vi "OE2011&OE2021_DATA Transmit.vi"(5 "Input Data":u8[](array[numeric])) -> (0 "Trig_Count":u8[](array[numeric]), 1 "PLL&Overload":T2, 2 "Parameter Values":T1, 3 "Total Date Array":dbl[][](array[numeric]), 4 "Buffer Count":u8)   [LabVIEW 2011]
panel:
  out "θh8":dbl[](array[numeric])
  out "Rh8":dbl[](array[numeric])
  out "θh7":dbl[](array[numeric])
  out "Rh7":dbl[](array[numeric])
  out "θh6":dbl[](array[numeric])
  out "Rh6":dbl[](array[numeric])
  out "θh5":dbl[](array[numeric])
  out "Rh5":dbl[](array[numeric])
  out "θh4":dbl[](array[numeric])
  out "Rh4":dbl[](array[numeric])
  out "θh3":dbl[](array[numeric])
  out "Rh3":dbl[](array[numeric])
  out "θh2":dbl[](array[numeric])
  out "Rh2":dbl[](array[numeric])
  out "θh1":dbl[](array[numeric])
  out "Rh1":dbl[](array[numeric])
  out "Osc1_Freq":dbl[](array[numeric])
  out "AUX IN2":dbl[](array[numeric])
  out "Yh8_Noise":dbl[](array[numeric])
  out "AUX IN1":dbl[](array[numeric])
  out "Osc2_Freq":dbl[](array[numeric])
  out "Xh8_Noise":dbl[](array[numeric])
  out "Yh6":dbl[](array[numeric])
  out "Yh5_Noise":dbl[](array[numeric])
  out "Xh6_Noise":dbl[](array[numeric])
  out "Yh6_Noise":dbl[](array[numeric])
  out "Xh7_Noise":dbl[](array[numeric])
  out "Yh7_Noise":dbl[](array[numeric])
  out "Xh6":dbl[](array[numeric])
  out "Xh7":dbl[](array[numeric])
  out "Yh7":dbl[](array[numeric])
  out "Xh8":dbl[](array[numeric])
  out "Yh8":dbl[](array[numeric])
  out "Xh1":dbl[](array[numeric])
  out "Yh1":dbl[](array[numeric])
  out "Xh2_Noise":dbl[](array[numeric])
  out "Xh2":dbl[](array[numeric])
  out "Yh2_Noise":dbl[](array[numeric])
  out "Xh3":dbl[](array[numeric])
  out "Yh3_Noise":dbl[](array[numeric])
  out "Xh4":dbl[](array[numeric])
  out "AUX IN3":dbl[](array[numeric])
  out "AUX IN4":dbl[](array[numeric])
  out "Yh4_Noise":dbl[](array[numeric])
  out "Xh5":dbl[](array[numeric])
  out "Yh2":dbl[](array[numeric])
  out "Xh1_Noise":dbl[](array[numeric])
  out "Yh1_Noise":dbl[](array[numeric])
  out "Yh3":dbl[](array[numeric])
  out "Xh3_Noise":dbl[](array[numeric])
  out "Yh4":dbl[](array[numeric])
  out "Xh4_Noise":dbl[](array[numeric])
  out "Yh5":dbl[](array[numeric])
  out "Xh5_Noise":dbl[](array[numeric])
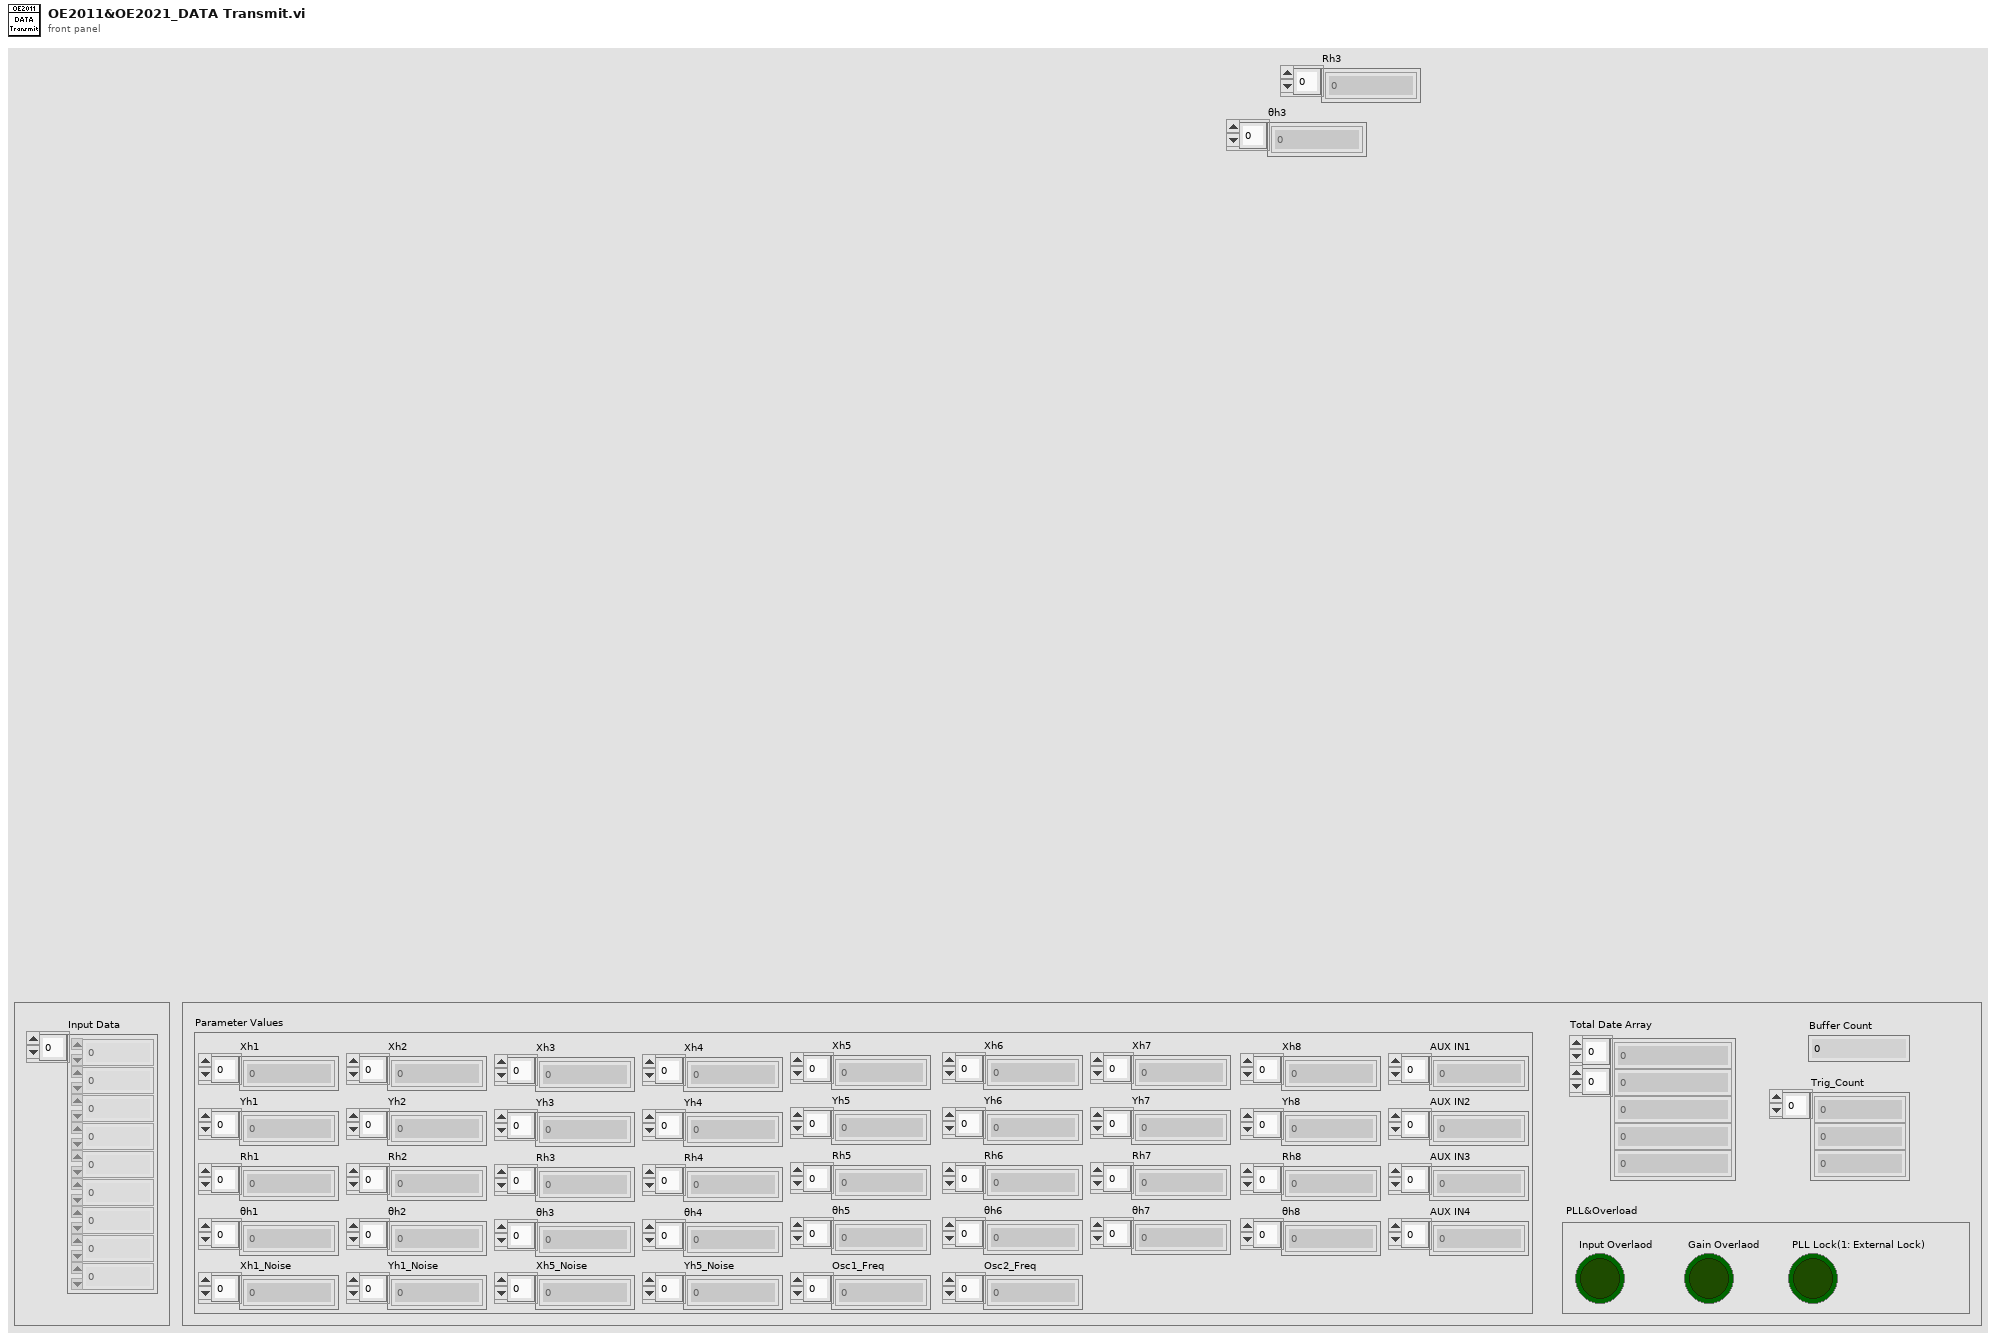
[diagram p1: front panel]
types:
  T1 = cluster{"Xh1":dbl[], "Yh1":dbl[], "Rh1":dbl[], "θh1":dbl[], "Xh1_Noise":dbl[], "Yh1_Noise":dbl[], "Xh2":dbl[], "Yh2":dbl[], "Rh2":dbl[], "θh2":dbl[], "Xh3":dbl[], "Yh3":dbl[], "Rh3":dbl[], "θh3":dbl[], "Xh4":dbl[], "Yh4":dbl[], "Rh4":dbl[], "θh4":dbl[], "Xh5":dbl[], "Yh5":dbl[], "Rh5":dbl[], "θh5":dbl[], "Xh5_Noise":dbl[], "Yh5_Noise":dbl[], "Xh6":dbl[], "Yh6":dbl[], "Rh6":dbl[], "θh6":dbl[], "Xh7":dbl[], "Yh7":dbl[], "Rh7":dbl[], "θh7":dbl[], "Xh8":dbl[], "Yh8":dbl[], "Rh8":dbl[], "θh8":dbl[], "Osc1_Freq":dbl[], "Osc2_Freq":dbl[], "AUX IN1":dbl[], "AUX IN2":dbl[], "AUX IN3":dbl[], "AUX IN4":dbl[]}
  T2 = cluster{"Input Overlaod":bool, "Gain Overlaod":bool, "PLL Lock(1: External Lock)":bool}
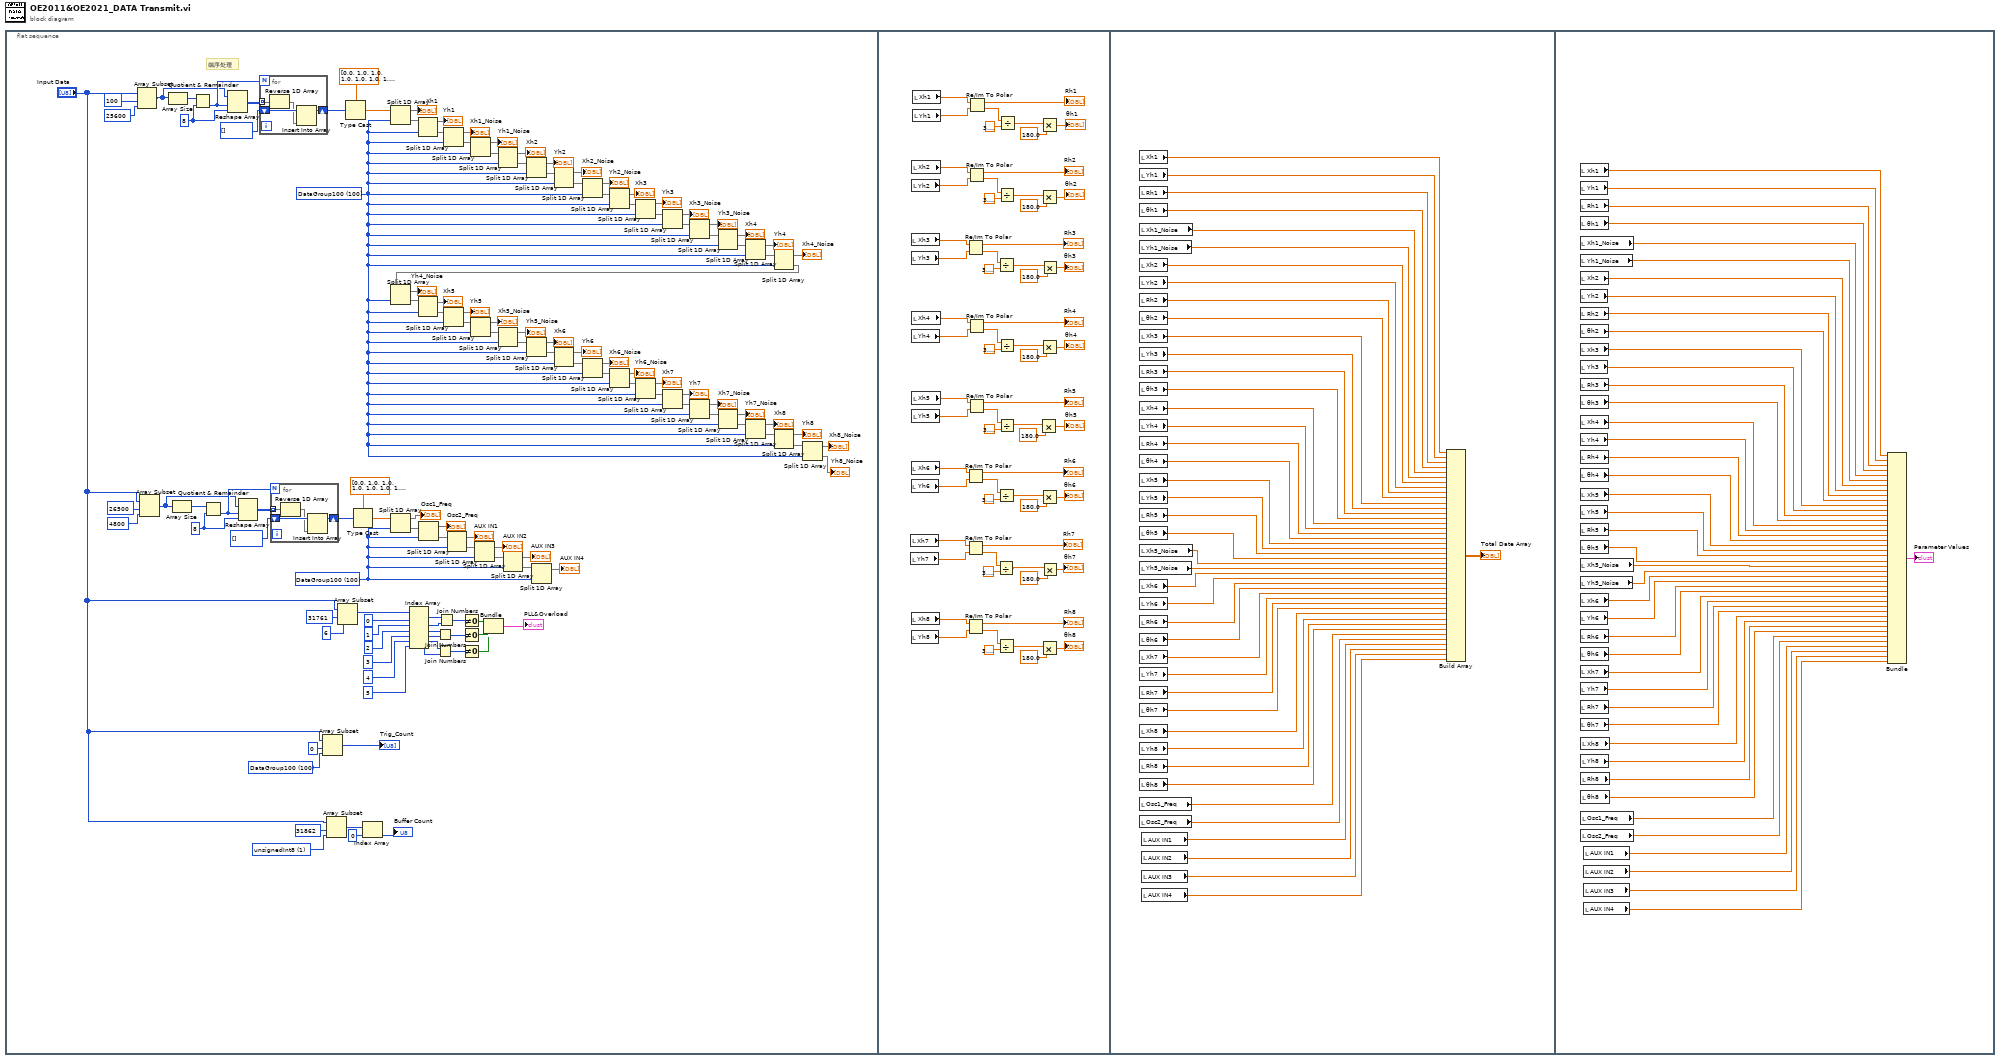
[diagram p0: block diagram]
diagram:
  n1 = flat-sequence {
    frame #0 {
      w5 = u16 1 items=["unsignedInt8"=1, "unsignedInt16"=2, "unsignedInt32"=4, "unsignedInt64"=8, "Float"=80, "Double"=160, "StartLength"=2240, "DataGroup50"=50, "DataGroup100"=100, "DataGroup20"=20] ("数据类型")
      w25 = 8 ("y")
      w30 = 8 ("y")
      w35 = u16 100 items=["unsignedInt8"=1, "unsignedInt16"=2, "unsignedInt32"=4, "unsignedInt64"=8, "Float"=80, "Double"=160, "StartLength"=2240, "DataGroup50"=50, "DataGroup100"=100, "DataGroup20"=20] ("数据类型")
      w46 = u16 100 items=["unsignedInt8"=1, "unsignedInt16"=2, "unsignedInt32"=4, "unsignedInt64"=8, "Float"=80, "Double"=160, "StartLength"=2240, "DataGroup50"=50, "DataGroup100"=100, "DataGroup20"=20] ("数据类型")
      w54 = u16 100 items=["unsignedInt8"=1, "unsignedInt16"=2, "unsignedInt32"=4, "unsignedInt64"=8, "Float"=80, "Double"=160, "StartLength"=2240, "DataGroup50"=50, "DataGroup100"=100, "DataGroup20"=20] ("数据类型")
      # "端序处理"
      n2 = Array Subset(array="Input Data", index=100 ("索引"), length=25600 ("长度")) -> (w22:u8[])
      n3 = Array Subset(array="Input Data", index=26500 ("索引"), length=4800 ("长度")) -> (w21:u8[])
      n4 = Array Size(array=w22) -> (size(s)=w29:i32)
      n5 = Array Size(array=w21) -> (size(s)=w24:i32)
      n6 = Quotient & Remainder(x=w29, y=w30) -> (floor(x/y)=w32:i32)  [unwired: 1 out]
      n7 = Quotient & Remainder(x=w24, y=w25) -> (floor(x/y)=w27:i32)  [unwired: 1 out]
      n8 = Reshape Array(w22, w32, w30) -> (w31:u8[][])
      n9 = Reshape Array(w21, w27, w25) -> (w26:u8[][])
      n10 = for {
        N: w32 -> [_]
        tunnel: w31 -> [w136] mode=indexing
        shift-right: [w134] -> w20
        shift-left: u8[] [] -> [w135]
        n11 = Reverse 1D Array(array=w136) -> (reversed array=w133:u8[])
        n12 = Insert Into Array(array=w135, new element=w133) -> (w134:u8[])  [unwired: 1 in]
      }
      n13 = for {
        N: w27 -> [_]
        tunnel: w26 -> [w132] mode=indexing
        shift-right: [w130] -> w23
        shift-left: u8[] [] -> [w131]
        n14 = Reverse 1D Array(array=w132) -> (reversed array=w129:u8[])
        n15 = Insert Into Array(array=w131, new element=w129) -> (w130:u8[])  [unwired: 1 in]
      }
      n16 = Array Subset(array="Input Data", index=0 ("索引"), length=w46) -> (→"Trig_Count":u8[])
      n17 = Array Subset(array="Input Data", index=31862 ("索引"), length=w5) -> (w3:u8[])
      n18 = Array Subset(array="Input Data", index=31761 ("索引"), length=6 ("长度")) -> (w51:u8[])
      n19 = Type Cast(type=dbl[] [0.0, 1.0, 1.0, 1.0, 1.0, 1.0, 1.0, 1.0, 1.0, 1.0, 1.0, 1.0, 1.0, 1.0, 1.0, 1.0, 1.0, 1.0, 1.0, 1.0, 1.0, 1.0, 1.0, 1.0, 1.0, 1.0, 1.0, 1.0, 1.0, 1.0, 1.0, 1.0, 1.0, 1.0, 1.0, 1.0, 1.0, 1.0, 1.0, 1.0, 1.0, 1.0, 1.0, 1.0, 1.0, 1.0, 1.0, 1.0, 1.0, 1.0, 1.0, 1.0, 1.0, 1.0, 1.0, 1.0, 1.0, 1.0, 1.0, 1.0, 1.0, 1.0, 1.0, 1.0, 1.0, 1.0, 1.0, 1.0, 1.0, 1.0, 1.0, 1.0, 1.0, 1.0, 1.0, 1.0, 1.0, 1.0, 1.0, 1.0, 1.0, 1.0, 1.0, 1.0, 1.0, 1.0, 1.0, 1.0, 1.0, 1.0, 1.0, 1.0, 1.0, 1.0, 1.0, 1.0, 1.0, 1.0, 1.0, 1.0, 1.0, 1.0, 1.0, 1.0, 1.0, 1.0, 1.0, 1.0, 1.0, 1.0, 1.0, 1.0, 1.0, 1.0, 1.0, 1.0, 1.0, 1.0, 1.0, 1.0, 1.0, 1.0, 1.0, 1.0, 1.0, 1.0, 1.0, 1.0, 1.0, 1.0, 1.0, 1.0, 1.0, 1.0, 1.0, 1.0, 1.0, 1.0, 1.0, 1.0, 1.0, 1.0, 1.0, 1.0, 1.0, 1.0, 1.0, 1.0, 1.0, 1.0, 1.0, 1.0, 1.0, 1.0, 1.0, 1.0, 1.0, 1.0, 1.0, 1.0, 1.0, 1.0, 1.0, 1.0, 1.0, 1.0, 1.0, 1.0, 1.0, 1.0, 1.0, 1.0, 1.0, 1.0, 1.0, 1.0, 1.0, 1.0, 1.0, 1.0, 1.0, 1.0, 1.0, 1.0, 1.0, 1.0, 1.0, 1.0, 1.0, 1.0, 1.0, 1.0, 1.0, 1.0, 1.0, 1.0, 1.0, 1.0, 1.0, 1.0, 1.0, 1.0, 1.0, 1.0, 1.0, 1.0, 1.0, 1.0, 1.0, 1.0, 1.0, 1.0, 1.0, 1.0, 1.0, 1.0, 1.0, 1.0, 1.0, 1.0, 1.0, 1.0, 1.0, 1.0, 1.0, 1.0, 1.0, 1.0, 1.0, 1.0, 1.0, 1.0, 1.0, 1.0, 1.0, 1.0, 1.0, 1.0, 1.0, 1.0, 1.0, 1.0, 1.0, 1.0, 1.0, 1.0, 1.0, 1.0, 1.0, 1.0, 1.0, 1.0, 1.0, 1.0, 1.0, 1.0, 1.0, 1.0, 1.0, 1.0, 1.0, 1.0, 1.0, 1.0, 1.0, 1.0, 1.0, 1.0, 1.0, 1.0, 1.0, 1.0, 1.0, 1.0, 1.0, 1.0, 1.0, 1.0, 1.0, 1.0, 1.0, 1.0, 1.0, 1.0, 1.0, 1.0, 1.0, 1.0, 1.0, 1.0, 1.0, 1.0, 1.0, 1.0, 1.0, 1.0, 1.0, 1.0, 1.0, 1.0, 1.0, 1.0, 1.0, 1.0, 1.0, 1.0, 1.0, 1.0, 1.0, 1.0, 1.0, 1.0, 1.0, 1.0, 1.0, 1.0, 1.0, 1.0, 1.0, 1.0, 1.0, 1.0, 1.0, 1.0, 1.0, 1.0, 1.0, 1.0, 1.0, 1.0, 1.0, 1.0, 1.0, 1.0, 1.0, 1.0, 1.0, 1.0, 1.0, 1.0, 1.0, 1.0, 1.0, 1.0, 1.0, 1.0, 1.0, 1.0, 1.0, 1.0, 1.0, 1.0, 1.0, 1.0, 1.0, 1.0, 1.0, 1.0, 1.0, 1.0, 1.0, 1.0, 1.0, 1.0, 1.0, 1.0, 1.0, 1.0, 1.0, 1.0, 1.0, 1.0, 1.0, 1.0, 1.0, 1.0, 1.0, 1.0, 1.0, 1.0, 1.0, 1.0, 1.0, 1.0, 1.0, 1.0, 1.0, 1.0, 1.0, 1.0, 1.0, 1.0, 1.0, 1.0, 1.0, 1.0, 1.0, 1.0, 1.0, 1.0, 0.0, 1.0, 1.0, 1.0, 1.0, 1.0, 1.0, 1.0, 1.0, 1.0, 1.0, 1.0, 1.0, 1.0, 1.0, 1.0, 1.0, 1.0, 1.0, 1.0, 1.0, 1.0, 1.0, 1.0, 1.0, 1.0, 1.0, 1.0, 1.0, 1.0, 1.0, 1.0, 1.0, 1.0, 1.0, 1.0, 1.0, 1.0, 1.0, 1.0, 1.0, 1.0, 1.0, 1.0, 1.0, 1.0, 1.0, 1.0, 1.0, 1.0, 1.0, 1.0, 1.0, 1.0, 1.0, 1.0, 1.0, 1.0, 1.0, 1.0, 1.0, 1.0, 1.0, 1.0, 1.0, 1.0, 1.0, 1.0, 1.0, 1.0, 1.0, 1.0, 1.0, 1.0, 1.0, 1.0, 1.0, 1.0, 1.0, 1.0, 1.0, 1.0, 1.0, 1.0, 1.0, 1.0, 1.0, 1.0, 1.0, 1.0, 1.0, 1.0, 1.0, 1.0, 1.0, 1.0, 1.0, 1.0, 1.0, 1.0, 1.0, 1.0, 1.0, 1.0, 1.0, 1.0, 1.0, 1.0, 1.0, 1.0, 1.0, 1.0, 1.0, 1.0, 1.0, 1.0, 1.0, 1.0, 1.0, 1.0, 1.0, 1.0, 1.0, 1.0, 1.0, 1.0, 1.0, 1.0, 1.0, 1.0, 1.0, 1.0, 1.0, 1.0, 1.0, 1.0, 1.0, 1.0, 1.0, 1.0, 1.0, 1.0, 1.0, 1.0, 1.0, 1.0, 1.0, 1.0, 1.0, 1.0, 1.0, 1.0, 1.0, 1.0, 1.0, 1.0, 1.0, 1.0, 1.0, 1.0, 1.0, 1.0, 1.0, 1.0, 1.0, 1.0, 1.0, 1.0, 1.0, 1.0, 1.0, 1.0, 1.0, 1.0, 1.0, 1.0, 1.0, 1.0, 1.0, 1.0, 1.0, 1.0, 1.0, 1.0, 1.0, 1.0, 1.0, 1.0, 1.0, 1.0, 1.0, 1.0, 1.0, 1.0, 1.0, 1.0, 1.0, 1.0, 1.0, 1.0, 1.0, 1.0, 1.0, 1.0, 1.0, 1.0, 1.0, 1.0, 1.0, 1.0, 1.0, 1.0, 1.0, 1.0, 1.0, 1.0, 1.0, 1.0, 1.0, 1.0, 1.0, 1.0, 1.0, 1.0, 1.0, 1.0, 1.0, 1.0, 1.0, 1.0, 1.0, 1.0, 1.0, 1.0, 1.0, 1.0, 1.0, 1.0, 1.0, 1.0, 1.0, 1.0, 1.0, 1.0, 1.0, 1.0, 1.0, 1.0, 1.0, 1.0, 1.0, 1.0, 1.0, 1.0, 1.0, 1.0, 1.0, 1.0, 1.0, 1.0, 1.0, 1.0, 1.0, 1.0, 1.0, 1.0, 1.0, 1.0, 1.0, 1.0, 1.0, 1.0, 1.0, 1.0, 1.0, 1.0, 1.0, 1.0, 1.0, 1.0, 1.0, 1.0, 1.0, 1.0, 1.0, 1.0, 1.0, 1.0, 1.0, 1.0, 1.0, 1.0, 1.0, 1.0, 1.0, 1.0, 1.0, 1.0, 1.0, 1.0, 1.0, 1.0, 1.0, 1.0, 1.0, 1.0, 1.0, 1.0, 1.0, 1.0, 1.0, 1.0, 1.0, 1.0, 1.0, 1.0, 1.0, 1.0, 1.0, 1.0, 1.0, 1.0, 1.0, 1.0, 1.0, 1.0, 1.0, 1.0, 1.0, 1.0, 1.0, 1.0, 1.0, 1.0, 1.0, 1.0, 1.0, 1.0, 1.0, 1.0, 1.0, 1.0, 1.0, 1.0, 1.0, 1.0, 1.0, 1.0, 1.0, 1.0, 1.0, 1.0, 1.0, 1.0, 1.0, 1.0, 1.0, 1.0, 1.0, 1.0, 1.0, 1.0, 1.0, 1.0, 1.0, 1.0, 1.0, 1.0, 1.0, 1.0, 1.0, 1.0, 1.0, 1.0, 1.0, 1.0, 1.0, 1.0, 1.0, 1.0, 1.0, 1.0, 1.0, 1.0, 1.0, 1.0, 1.0, 1.0, 1.0, 1.0, 1.0, 1.0, 1.0, 1.0, 1.0, 1.0, 1.0, 1.0, 1.0, 1.0], x=w20) -> (*(type *) &x=w125:dbl[])
      n20 = Type Cast(type=dbl[] [0.0, 1.0, 1.0, 1.0, 1.0, 1.0, 1.0, 1.0, 1.0, 1.0, 1.0, 1.0, 1.0, 1.0, 1.0, 1.0, 1.0, 1.0, 1.0, 1.0, 1.0, 1.0, 1.0, 1.0, 1.0, 1.0, 1.0, 1.0, 1.0, 1.0, 1.0, 1.0, 1.0, 1.0, 1.0, 1.0, 1.0, 1.0, 1.0, 1.0, 1.0, 1.0, 1.0, 1.0, 1.0, 1.0, 1.0, 1.0, 1.0, 1.0, 1.0, 1.0, 1.0, 1.0, 1.0, 1.0, 1.0, 1.0, 1.0, 1.0, 1.0, 1.0, 1.0, 1.0, 1.0, 1.0, 1.0, 1.0, 1.0, 1.0, 1.0, 1.0, 1.0, 1.0, 1.0, 1.0, 1.0, 1.0, 1.0, 1.0, 1.0, 1.0, 1.0, 1.0, 1.0, 1.0, 1.0, 1.0, 1.0, 1.0, 1.0, 1.0, 1.0, 1.0, 1.0, 1.0, 1.0, 1.0, 1.0, 1.0, 1.0, 1.0, 1.0, 1.0, 1.0, 1.0, 1.0, 1.0, 1.0, 1.0, 1.0, 1.0, 1.0, 1.0, 1.0, 1.0, 1.0, 1.0, 1.0, 1.0, 1.0, 1.0, 1.0, 1.0, 1.0, 1.0, 1.0, 1.0, 1.0, 1.0, 1.0, 1.0, 1.0, 1.0, 1.0, 1.0, 1.0, 1.0, 1.0, 1.0, 1.0, 1.0, 1.0, 1.0, 1.0, 1.0, 1.0, 1.0, 1.0, 1.0, 1.0, 1.0, 1.0, 1.0, 1.0, 1.0, 1.0, 1.0, 1.0, 1.0, 1.0, 1.0, 1.0, 1.0, 1.0, 1.0, 1.0, 1.0, 1.0, 1.0, 1.0, 1.0, 1.0, 1.0, 1.0, 1.0, 1.0, 1.0, 1.0, 1.0, 1.0, 1.0, 1.0, 1.0, 1.0, 1.0, 1.0, 1.0, 1.0, 1.0, 1.0, 1.0, 1.0, 1.0, 1.0, 1.0, 1.0, 1.0, 1.0, 1.0, 1.0, 1.0, 1.0, 1.0, 1.0, 1.0, 1.0, 1.0, 1.0, 1.0, 1.0, 1.0, 1.0, 1.0, 1.0, 1.0, 1.0, 1.0, 1.0, 1.0, 1.0, 1.0, 1.0, 1.0, 1.0, 1.0, 1.0, 1.0, 1.0, 1.0, 1.0, 1.0, 1.0, 1.0, 1.0, 1.0, 1.0, 1.0, 1.0, 1.0, 1.0, 1.0, 1.0, 1.0, 1.0, 1.0, 1.0, 1.0, 1.0, 1.0, 1.0, 1.0, 1.0, 1.0, 1.0, 1.0, 1.0, 1.0, 1.0, 1.0, 1.0, 1.0, 1.0, 1.0, 1.0, 1.0, 1.0, 1.0, 1.0, 1.0, 1.0, 1.0, 1.0, 1.0, 1.0, 1.0, 1.0, 1.0, 1.0, 1.0, 1.0, 1.0, 1.0, 1.0, 1.0, 1.0, 1.0, 1.0, 1.0, 1.0, 1.0, 1.0, 1.0, 1.0, 1.0, 1.0, 1.0, 1.0, 1.0, 1.0, 1.0, 1.0, 1.0, 1.0, 1.0, 1.0, 1.0, 1.0, 1.0, 1.0, 1.0, 1.0, 1.0, 1.0, 1.0, 1.0, 1.0, 1.0, 1.0, 1.0, 1.0, 1.0, 1.0, 1.0, 1.0, 1.0, 1.0, 1.0, 1.0, 1.0, 1.0, 1.0, 1.0, 1.0, 1.0, 1.0, 1.0, 1.0, 1.0, 1.0, 1.0, 1.0, 1.0, 1.0, 1.0, 1.0, 1.0, 1.0, 1.0, 1.0, 1.0, 1.0, 1.0, 1.0, 1.0, 1.0, 1.0, 1.0, 1.0, 1.0, 1.0, 1.0, 1.0, 1.0, 1.0, 1.0, 1.0, 1.0, 1.0, 1.0, 1.0, 1.0, 1.0, 1.0, 1.0, 1.0, 1.0, 1.0, 1.0, 1.0, 1.0, 1.0, 1.0, 1.0, 1.0, 1.0, 1.0, 1.0, 1.0, 1.0, 1.0, 1.0, 1.0, 1.0, 1.0, 1.0, 1.0, 1.0, 1.0, 1.0, 0.0, 1.0, 1.0, 1.0, 1.0, 1.0, 1.0, 1.0, 1.0, 1.0, 1.0, 1.0, 1.0, 1.0, 1.0, 1.0, 1.0, 1.0, 1.0, 1.0, 1.0, 1.0, 1.0, 1.0, 1.0, 1.0, 1.0, 1.0, 1.0, 1.0, 1.0, 1.0, 1.0, 1.0, 1.0, 1.0, 1.0, 1.0, 1.0, 1.0, 1.0, 1.0, 1.0, 1.0, 1.0, 1.0, 1.0, 1.0, 1.0, 1.0, 1.0, 1.0, 1.0, 1.0, 1.0, 1.0, 1.0, 1.0, 1.0, 1.0, 1.0, 1.0, 1.0, 1.0, 1.0, 1.0, 1.0, 1.0, 1.0, 1.0, 1.0, 1.0, 1.0, 1.0, 1.0, 1.0, 1.0, 1.0, 1.0, 1.0, 1.0, 1.0, 1.0, 1.0, 1.0, 1.0, 1.0, 1.0, 1.0, 1.0, 1.0, 1.0, 1.0, 1.0, 1.0, 1.0, 1.0, 1.0, 1.0, 1.0, 1.0, 1.0, 1.0, 1.0, 1.0, 1.0, 1.0, 1.0, 1.0, 1.0, 1.0, 1.0, 1.0, 1.0, 1.0, 1.0, 1.0, 1.0, 1.0, 1.0, 1.0, 1.0, 1.0, 1.0, 1.0, 1.0, 1.0, 1.0, 1.0, 1.0, 1.0, 1.0, 1.0, 1.0, 1.0, 1.0, 1.0, 1.0, 1.0, 1.0, 1.0, 1.0, 1.0, 1.0, 1.0, 1.0, 1.0, 1.0, 1.0, 1.0, 1.0, 1.0, 1.0, 1.0, 1.0, 1.0, 1.0, 1.0, 1.0, 1.0, 1.0, 1.0, 1.0, 1.0, 1.0, 1.0, 1.0, 1.0, 1.0, 1.0, 1.0, 1.0, 1.0, 1.0, 1.0, 1.0, 1.0, 1.0, 1.0, 1.0, 1.0, 1.0, 1.0, 1.0, 1.0, 1.0, 1.0, 1.0, 1.0, 1.0, 1.0, 1.0, 1.0, 1.0, 1.0, 1.0, 1.0, 1.0, 1.0, 1.0, 1.0, 1.0, 1.0, 1.0, 1.0, 1.0, 1.0, 1.0, 1.0, 1.0, 1.0, 1.0, 1.0, 1.0, 1.0, 1.0, 1.0, 1.0, 1.0, 1.0, 1.0, 1.0, 1.0, 1.0, 1.0, 1.0, 1.0, 1.0, 1.0, 1.0, 1.0, 1.0, 1.0, 1.0, 1.0, 1.0, 1.0, 1.0, 1.0, 1.0, 1.0, 1.0, 1.0, 1.0, 1.0, 1.0, 1.0, 1.0, 1.0, 1.0, 1.0, 1.0, 1.0, 1.0, 1.0, 1.0, 1.0, 1.0, 1.0, 1.0, 1.0, 1.0, 1.0, 1.0, 1.0, 1.0, 1.0, 1.0, 1.0, 1.0, 1.0, 1.0, 1.0, 1.0, 1.0, 1.0, 1.0, 1.0, 1.0, 1.0, 1.0, 1.0, 1.0, 1.0, 1.0, 1.0, 1.0, 1.0, 1.0, 1.0, 1.0, 1.0, 1.0, 1.0, 1.0, 1.0, 1.0, 1.0, 1.0, 1.0, 1.0, 1.0, 1.0, 1.0, 1.0, 1.0, 1.0, 1.0, 1.0, 1.0, 1.0, 1.0, 1.0, 1.0, 1.0, 1.0, 1.0, 1.0, 1.0, 1.0, 1.0, 1.0, 1.0, 1.0, 1.0, 1.0, 1.0, 1.0, 1.0, 1.0, 1.0, 1.0, 1.0, 1.0, 1.0, 1.0, 1.0, 1.0, 1.0, 1.0, 1.0, 1.0, 1.0, 1.0, 1.0, 1.0, 1.0, 1.0, 1.0, 1.0, 1.0, 1.0, 1.0, 1.0, 1.0, 1.0, 1.0, 1.0, 1.0, 1.0, 1.0, 1.0, 1.0, 1.0, 1.0, 1.0, 1.0, 1.0, 1.0, 1.0, 1.0, 1.0, 1.0, 1.0, 1.0, 1.0, 1.0, 1.0, 1.0, 1.0, 1.0, 1.0, 1.0, 1.0, 1.0, 1.0, 1.0, 1.0, 1.0, 1.0, 1.0, 1.0, 1.0, 1.0, 1.0, 1.0, 1.0, 1.0, 1.0, 1.0], x=w23) -> (*(type *) &x=w37:dbl[])
      n21 = Index Array(array=w3, index=0 ("索引")) -> (element=→"Buffer Count":u8)
      n22 = Split 1D Array(array=w125, index=w54) -> (first subarray=→"Xh1":dbl[], second subarray=w126:dbl[])
      n23 = Split 1D Array(array=w37, index=w35) -> (first subarray=→"Osc1_Freq":dbl[], second subarray=w55:dbl[])
      n24 = Index Array(array=w51, index #1=0 ("索引"), index #2=1 ("索引"), index #3=2 ("索引"), index #4=3 ("索引"), index #5=4 ("索引"), index #6=5 ("索引")) -> (element #1=w14:u8, element #2=w15:u8, element #3=w11:u8, element #4=w10:u8, element #5=w9:u8, element #6=w8:u8)
      n25 = Split 1D Array(array=w126, index=w54) -> (first subarray=→"Yh1":dbl[], second subarray=w127:dbl[])
      n26 = Split 1D Array(array=w55, index=w35) -> (first subarray=→"Osc2_Freq":dbl[], second subarray=w61:dbl[])
      n27 = Join Numbers(hi=w11, lo=w10) -> ((hi.lo)=w12:u16)
      n28 = Join Numbers(hi=w9, lo=w8) -> ((hi.lo)=w7:u16)
      n29 = Join Numbers(hi=w14, lo=w15) -> ((hi.lo)=w13:u16)
      n30 = Split 1D Array(array=w127, index=w54) -> (first subarray=→"Xh1_Noise":dbl[], second subarray=w118:dbl[])
      n31 = Split 1D Array(array=w61, index=w35) -> (first subarray=→"AUX IN1":dbl[], second subarray=w59:dbl[])
      n32 = Not Equal To 0?(x=w13) -> (x != 0?=w43:bool)
      n33 = Not Equal To 0?(x=w12) -> (x != 0?=w42:bool)
      n34 = Not Equal To 0?(x=w7) -> (x != 0?=w41:bool)
      n35 = Split 1D Array(array=w118, index=w54) -> (first subarray=→"Yh1_Noise":dbl[], second subarray=w120:dbl[])
      n36 = Split 1D Array(array=w59, index=w35) -> (first subarray=→"AUX IN2":dbl[], second subarray=w60:dbl[])
      n37 = Bundle(w43, w42, w41) -> (→"PLL&Overload":cluster{bool, bool, bool})  [unwired: 1 in]
      n38 = Split 1D Array(array=w120, index=w54) -> (first subarray=→"Xh2":dbl[], second subarray=w119:dbl[])
      n39 = Split 1D Array(array=w60, index=w35) -> (first subarray=→"AUX IN3":dbl[], second subarray=w58:dbl[])
      n40 = Split 1D Array(array=w119, index=w54) -> (first subarray=→"Yh2":dbl[], second subarray=w113:dbl[])
      n41 = Split 1D Array(array=w58, index=w35) -> (first subarray=→"AUX IN4":dbl[])  [unwired: 1 out]
      n42 = Split 1D Array(array=w113, index=w54) -> (first subarray=→"Xh2_Noise":dbl[], second subarray=w111:dbl[])
      n43 = Split 1D Array(array=w111, index=w54) -> (first subarray=→"Yh2_Noise":dbl[], second subarray=w110:dbl[])
      n44 = Split 1D Array(array=w110, index=w54) -> (first subarray=→"Xh3":dbl[], second subarray=w109:dbl[])
      n45 = Split 1D Array(array=w109, index=w54) -> (first subarray=→"Yh3":dbl[], second subarray=w105:dbl[])
      n46 = Split 1D Array(array=w105, index=w54) -> (first subarray=→"Xh3_Noise":dbl[], second subarray=w103:dbl[])
      n47 = Split 1D Array(array=w103, index=w54) -> (first subarray=→"Yh3_Noise":dbl[], second subarray=w101:dbl[])
      n48 = Split 1D Array(array=w101, index=w54) -> (first subarray=→"Xh4":dbl[], second subarray=w128:dbl[])
      n49 = Split 1D Array(array=w128, index=w54) -> (first subarray=→"Yh4":dbl[], second subarray=w121:dbl[])
      n50 = Split 1D Array(array=w121, index=w54) -> (first subarray=→"Xh4_Noise":dbl[], second subarray=w71:dbl[])
      n51 = Split 1D Array(array=w71, index=w54) -> (first subarray=→"Yh4_Noise":dbl[], second subarray=w74:dbl[])
      n52 = Split 1D Array(array=w74, index=w54) -> (first subarray=→"Xh5":dbl[], second subarray=w73:dbl[])
      n53 = Split 1D Array(array=w73, index=w54) -> (first subarray=→"Yh5":dbl[], second subarray=w78:dbl[])
      n54 = Split 1D Array(array=w78, index=w54) -> (first subarray=→"Xh5_Noise":dbl[], second subarray=w76:dbl[])
      n55 = Split 1D Array(array=w76, index=w54) -> (first subarray=→"Yh5_Noise":dbl[], second subarray=w77:dbl[])
      n56 = Split 1D Array(array=w77, index=w54) -> (first subarray=→"Xh6":dbl[], second subarray=w80:dbl[])
      n57 = Split 1D Array(array=w80, index=w54) -> (first subarray=→"Yh6":dbl[], second subarray=w82:dbl[])
      n58 = Split 1D Array(array=w82, index=w54) -> (first subarray=→"Xh6_Noise":dbl[], second subarray=w83:dbl[])
      n59 = Split 1D Array(array=w83, index=w54) -> (first subarray=→"Yh6_Noise":dbl[], second subarray=w84:dbl[])
      n60 = Split 1D Array(array=w84, index=w54) -> (first subarray=→"Xh7":dbl[], second subarray=w88:dbl[])
      n61 = Split 1D Array(array=w88, index=w54) -> (first subarray=→"Yh7":dbl[], second subarray=w90:dbl[])
      n62 = Split 1D Array(array=w90, index=w54) -> (first subarray=→"Xh7_Noise":dbl[], second subarray=w92:dbl[])
      n63 = Split 1D Array(array=w92, index=w54) -> (first subarray=→"Yh7_Noise":dbl[], second subarray=w72:dbl[])
      n64 = Split 1D Array(array=w72, index=w54) -> (first subarray=→"Xh8":dbl[], second subarray=w75:dbl[])
      n65 = Split 1D Array(array=w75, index=w54) -> (first subarray=→"Yh8":dbl[], second subarray=w66:dbl[])
      n66 = Split 1D Array(array=w66, index=w54) -> (first subarray=→"Xh8_Noise":dbl[], second subarray=→"Yh8_Noise":dbl[])
    }
    frame #1 {
      n67 = local read "Xh7"() -> (w175:dbl[])
      n68 = local read "Yh7"() -> (w174:dbl[])
      n69 = local read "Xh3"() -> (w186:dbl[])
      n70 = local read "Yh3"() -> (w187:dbl[])
      n71 = local read "Xh6"() -> (w170:dbl[])
      n72 = local read "Yh6"() -> (w169:dbl[])
      n73 = local read "Xh8"() -> (w180:dbl[])
      n74 = local read "Yh8"() -> (w179:dbl[])
      n75 = local read "Xh2"() -> (w191:dbl[])
      n76 = local read "Yh2"() -> (w192:dbl[])
      n77 = local read "Xh4"() -> (w181:dbl[])
      n78 = local read "Yh4"() -> (w182:dbl[])
      n79 = local read "Xh5"() -> (w161:dbl[])
      n80 = local read "Yh5"() -> (w162:dbl[])
      n81 = local read "Xh1"() -> (w200:dbl[])
      n82 = local read "Yh1"() -> (w199:dbl[])
      n83 = Re/Im To Polar(2:w174, 3:w175) -> (0:w172:dbl[], 1:→"Rh7":dbl[])
      n84 = Re/Im To Polar(2:w187, 3:w186) -> (0:w189:dbl[], 1:→"Rh3":dbl[])
      n85 = Re/Im To Polar(2:w169, 3:w170) -> (0:w167:dbl[], 1:→"Rh6":dbl[])
      n86 = Re/Im To Polar(2:w179, 3:w180) -> (0:w177:dbl[], 1:→"Rh8":dbl[])
      n87 = Re/Im To Polar(2:w192, 3:w191) -> (0:w194:dbl[], 1:→"Rh2":dbl[])
      n88 = Re/Im To Polar(2:w182, 3:w181) -> (0:w184:dbl[], 1:→"Rh4":dbl[])
      n89 = Re/Im To Polar(2:w162, 3:w161) -> (0:w164:dbl[], 1:→"Rh5":dbl[])
      n90 = Re/Im To Polar(2:w199, 3:w200) -> (0:w197:dbl[], 1:→"Rh1":dbl[])
      n91 = Divide(x=w172, y=3.141592653589793) -> (x/y=w145:dbl[])
      n92 = Divide(x=w189, y=3.141592653589793) -> (x/y=w138:dbl[])
      n93 = Divide(x=w167, y=3.141592653589793) -> (x/y=w144:dbl[])
      n94 = Divide(x=w177, y=3.141592653589793) -> (x/y=w147:dbl[])
      n95 = Divide(x=w194, y=3.141592653589793) -> (x/y=w155:dbl[])
      n96 = Divide(x=w184, y=3.141592653589793) -> (x/y=w139:dbl[])
      n97 = Divide(x=w164, y=3.141592653589793) -> (x/y=w142:dbl[])
      n98 = Divide(x=w197, y=3.141592653589793) -> (x/y=w159:dbl[])
      n99 = Multiply(x=w142, y=180.0) -> (x*y=→"θh5":dbl[])
      n100 = Multiply(x=w159, y=180.0) -> (x*y=→"θh1":dbl[])
      n101 = Multiply(x=w155, y=180.0) -> (x*y=→"θh2":dbl[])
      n102 = Multiply(x=w139, y=180.0) -> (x*y=→"θh4":dbl[])
      n103 = Multiply(x=w144, y=180.0) -> (x*y=→"θh6":dbl[])
      n104 = Multiply(x=w147, y=180.0) -> (x*y=→"θh8":dbl[])
      n105 = Multiply(x=w138, y=180.0) -> (x*y=→"θh3":dbl[])
      n106 = Multiply(x=w145, y=180.0) -> (x*y=→"θh7":dbl[])
    }
    frame #2 {
      n107 = local read "Xh1"() -> (w243:dbl[])
      n108 = local read "Yh1"() -> (w242:dbl[])
      n109 = local read "Rh1"() -> (w241:dbl[])
      n110 = local read "θh1"() -> (w240:dbl[])
      n111 = local read "Xh1_Noise"() -> (w239:dbl[])
      n112 = local read "Yh1_Noise"() -> (w238:dbl[])
      n113 = local read "Xh2"() -> (w237:dbl[])
      n114 = local read "Yh2"() -> (w236:dbl[])
      n115 = local read "Rh2"() -> (w235:dbl[])
      n116 = local read "θh2"() -> (w234:dbl[])
      n117 = local read "Xh3"() -> (w220:dbl[])
      n118 = local read "Yh3"() -> (w219:dbl[])
      n119 = local read "Rh3"() -> (w218:dbl[])
      n120 = local read "θh3"() -> (w217:dbl[])
      n121 = local read "Xh4"() -> (w233:dbl[])
      n122 = local read "Yh4"() -> (w232:dbl[])
      n123 = local read "Rh4"() -> (w231:dbl[])
      n124 = local read "θh4"() -> (w230:dbl[])
      n125 = local read "Xh5"() -> (w229:dbl[])
      n126 = local read "Yh5"() -> (w228:dbl[])
      n127 = local read "Rh5"() -> (w227:dbl[])
      n128 = local read "θh5"() -> (w226:dbl[])
      n129 = local read "Xh5_Noise"() -> (w225:dbl[])
      n130 = local read "Yh5_Noise"() -> (w224:dbl[])
      n131 = local read "Xh6"() -> (w223:dbl[])
      n132 = local read "Yh6"() -> (w222:dbl[])
      n133 = local read "Rh6"() -> (w216:dbl[])
      n134 = local read "θh6"() -> (w215:dbl[])
      n135 = local read "Xh7"() -> (w221:dbl[])
      n136 = local read "Yh7"() -> (w213:dbl[])
      n137 = local read "Rh7"() -> (w212:dbl[])
      n138 = local read "θh7"() -> (w211:dbl[])
      n139 = local read "Xh8"() -> (w210:dbl[])
      n140 = local read "Yh8"() -> (w209:dbl[])
      n141 = local read "Rh8"() -> (w208:dbl[])
      n142 = local read "θh8"() -> (w207:dbl[])
      n143 = local read "Osc1_Freq"() -> (w206:dbl[])
      n144 = local read "Osc2_Freq"() -> (w205:dbl[])
      n145 = local read "AUX IN1"() -> (w204:dbl[])
      n146 = local read "AUX IN2"() -> (w203:dbl[])
      n147 = local read "AUX IN3"() -> (w202:dbl[])
      n148 = local read "AUX IN4"() -> (w201:dbl[])
      n149 = Build Array(w243, w242, w241, w240, w239, w238, w237, w236, w235, w234, w220, w219, w218, w217, w233, w232, w231, w230, w229, w228, w227, w226, w225, w224, w223, w222, w216, w215, w221, w213, w212, w211, w210, w209, w208, w207, w206, w205, w204, w203, w202, w201) -> (→"Total Date Array":dbl[][])
    }
    frame #3 {
      n150 = local read "Xh1"() -> (w286:dbl[])
      n151 = local read "Yh1"() -> (w285:dbl[])
      n152 = local read "Rh1"() -> (w284:dbl[])
      n153 = local read "θh1"() -> (w283:dbl[])
      n154 = local read "Xh1_Noise"() -> (w282:dbl[])
      n155 = local read "Yh1_Noise"() -> (w281:dbl[])
      n156 = local read "Xh2"() -> (w280:dbl[])
      n157 = local read "Yh2"() -> (w279:dbl[])
      n158 = local read "Rh2"() -> (w278:dbl[])
      n159 = local read "θh2"() -> (w277:dbl[])
      n160 = local read "Xh3"() -> (w263:dbl[])
      n161 = local read "Yh3"() -> (w262:dbl[])
      n162 = local read "Rh3"() -> (w261:dbl[])
      n163 = local read "θh3"() -> (w260:dbl[])
      n164 = local read "Xh4"() -> (w276:dbl[])
      n165 = local read "Yh4"() -> (w275:dbl[])
      n166 = local read "Rh4"() -> (w274:dbl[])
      n167 = local read "θh4"() -> (w273:dbl[])
      n168 = local read "Xh5"() -> (w272:dbl[])
      n169 = local read "Yh5"() -> (w271:dbl[])
      n170 = local read "Rh5"() -> (w270:dbl[])
      n171 = local read "θh5"() -> (w269:dbl[])
      n172 = local read "Xh5_Noise"() -> (w268:dbl[])
      n173 = local read "Yh5_Noise"() -> (w267:dbl[])
      n174 = local read "Xh6"() -> (w266:dbl[])
      n175 = local read "Yh6"() -> (w265:dbl[])
      n176 = local read "Rh6"() -> (w259:dbl[])
      n177 = local read "θh6"() -> (w258:dbl[])
      n178 = local read "Xh7"() -> (w264:dbl[])
      n179 = local read "Yh7"() -> (w257:dbl[])
      n180 = local read "Rh7"() -> (w256:dbl[])
      n181 = local read "θh7"() -> (w255:dbl[])
      n182 = local read "Xh8"() -> (w254:dbl[])
      n183 = local read "Yh8"() -> (w253:dbl[])
      n184 = local read "Rh8"() -> (w252:dbl[])
      n185 = local read "θh8"() -> (w251:dbl[])
      n186 = local read "Osc1_Freq"() -> (w250:dbl[])
      n187 = local read "Osc2_Freq"() -> (w249:dbl[])
      n188 = local read "AUX IN1"() -> (w248:dbl[])
      n189 = local read "AUX IN2"() -> (w247:dbl[])
      n190 = local read "AUX IN3"() -> (w246:dbl[])
      n191 = local read "AUX IN4"() -> (w245:dbl[])
      n192 = Bundle("Xh1"=w286, "Yh1"=w285, "Rh1"=w284, "θh1"=w283, "Xh1_Noise"=w282, "Yh1_Noise"=w281, "Xh2"=w280, "Yh2"=w279, "Rh2"=w278, "θh2"=w277, "Xh3"=w263, "Yh3"=w262, "Rh3"=w261, "θh3"=w260, "Xh4"=w276, "Yh4"=w275, "Rh4"=w274, "θh4"=w273, "Xh5"=w272, "Yh5"=w271, "Rh5"=w270, "θh5"=w269, "Xh5_Noise"=w268, "Yh5_Noise"=w267, "Xh6"=w266, "Yh6"=w265, "Rh6"=w259, "θh6"=w258, "Xh7"=w264, "Yh7"=w257, "Rh7"=w256, "θh7"=w255, "Xh8"=w254, "Yh8"=w253, "Rh8"=w252, "θh8"=w251, "Osc1_Freq"=w250, "Osc2_Freq"=w249, "AUX IN1"=w248, "AUX IN2"=w247, "AUX IN3"=w246, "AUX IN4"=w245) -> (→"Parameter Values":T1)  [unwired: 1 in]
    }
  }
